vi "Configure Display Priority.vi"(8 "error in (no error)":errorcluster, 10 "Priority (0)":T1(ring), 11 "VISA resource name":refnum<visa-resource-name>) -> (0 "error out":errorcluster, 3 "VISA resource name out":refnum<visa-resource-name>)   [LabVIEW 2013, in "LeCroy Wave Series.lvlib"]
doc: "Sets the optimizer slider for the performance between Analysis and Display, and also provides the option to disable or enable the display. For highest throughput, set the priority to Analysis or to Disable Display. \n\nWarning - if you choose to disable the display, be sure to re-enable it when exiting your application."
uses:
  LeCroy Wave Series.lvlib
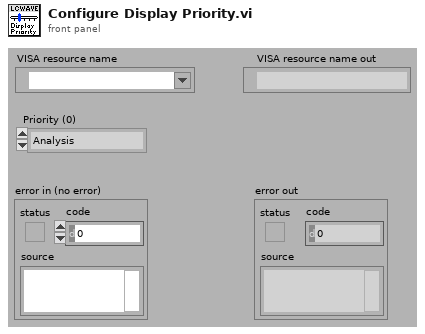
[diagram p1: front panel]
types:
  T1 = enum16{"Analysis", "AnalysisMid", "Default", "DisplayMid", "Display", "Disable Display", "Enable Display"}
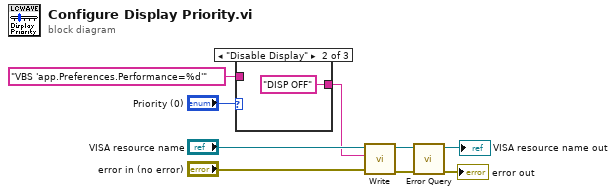
[diagram p0: block diagram]
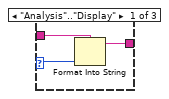
[diagram p2: hidden frame]
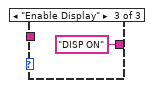
[diagram p3: hidden frame]
diagram:
  n1 = case shown="\"Disable Display\"" "Priority (0)" {
    selector: "Priority (0)" -> [w10 _ _]
    tunnel: "VBS 'app.Preferences.Performance=%d'" ("format string") -> [w12 _ _]
    tunnel: [w11 "DISP OFF" "DISP ON"] -> w4
    frame "Analysis".."Display" {
      n2 = Format Into String(format string=w12, w10) -> (resulting string=w11:string)  [unwired: 2 in, 1 out]
    }
    frame "Disable Display" {
    }
    frame "Enable Display" {
    }
  }
  n3 = call "Write.vi"("error in (no error)"="error in (no error)", "Write Buffer"=w4, "VISA resource name"="VISA resource name") -> ("error out"=w2:errorcluster, "VISA resource name out"=w1:refnum<visa-resource-name>)  [unwired: 6 in, 1 out]
  n4 = call "Error Query.vi"("error in (no error)"=w2, "VISA resource name"=w1) -> ("error out"=→"error out":errorcluster, "VISA resource name out"=→"VISA resource name out":refnum<visa-resource-name>)  [unwired: 6 in, 2 out]
